vi "ISX3_Parse_Data.vi"(0 "Array":u8[](array[numeric])) -> (1 "Row ID":u16, 2 "Real":sgl, 3 "Imag":sgl)   [LabVIEW 2012, in "Sciospec ISX3 Impedance Analyzer.lvlib"]
uses:
  Sciospec ISX3 Impedance Analyzer.lvlib
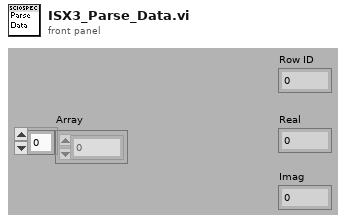
[diagram p1: front panel]
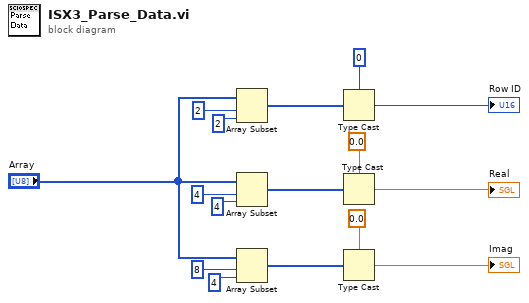
[diagram p0: block diagram]
diagram:
  n1 = Array Subset(array="Array", index=2 ("Index"), length=2 ("Länge")) -> (w15:u8[])
  n2 = Array Subset(array="Array", index=4 ("Index"), length=4 ("Länge")) -> (w10:u8[])
  n3 = Array Subset(array="Array", index=8 ("Index"), length=4 ("Länge")) -> (w2:u8[])
  n4 = Type Cast(type=u16 0, x=w15) -> (*(type *) &x=→"Row ID":u16)
  n5 = Type Cast(type=sgl 0.0, x=w10) -> (*(type *) &x=→"Real":sgl)
  n6 = Type Cast(type=sgl 0.0, x=w2) -> (*(type *) &x=→"Imag":sgl)
